vi "ACT_6_Task3_825005609.vi"() -> ()   [LabVIEW 2016]
panel:
  out "Numeric 2":dbl
  in  "n is":u32
  in  "x is.":u32
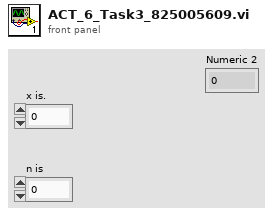
[diagram p1: front panel]
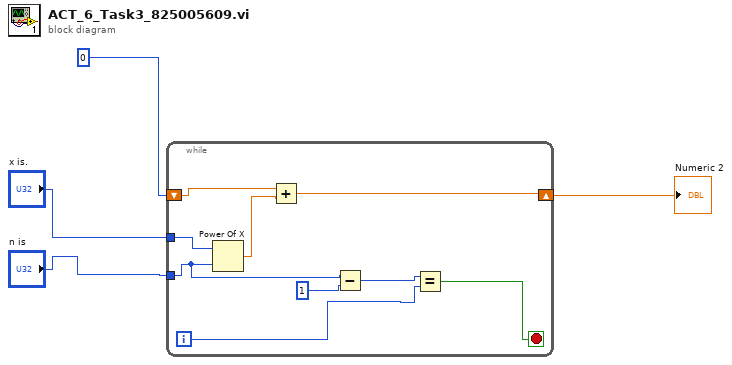
[diagram p0: block diagram]
diagram:
  n1 = while {
    tunnel: "x is." -> [w13]
    tunnel: "n is" -> [w11]
    shift-right: [w6] -> w1
    shift-left: 0 -> [w5]
    i -> [w7]
    stop <- w8 stop-if-true
    n2 = Power Of X(1:w11, 2:w13) -> (0:w12:dbl)
    n3 = Add(x=w5, y=w12) -> (x+y=w6:dbl)
    n4 = Subtract(x=w11, y=1) -> (x-y=w9:u32)
    n5 = Equal?(x=w9, y=w7) -> (x = y?=w8:bool)
  }
  "Numeric 2" <- w1
